vi "Evaluate Method Status.vi"(11 "Results":T2[](array[typedef])) -> (3 "Status":T1)   [LabVIEW 2020, in "Result.lvlib"]
uses:
  Result.lvlib
  Result.ctl
  Status.ctl
  Type.ctl
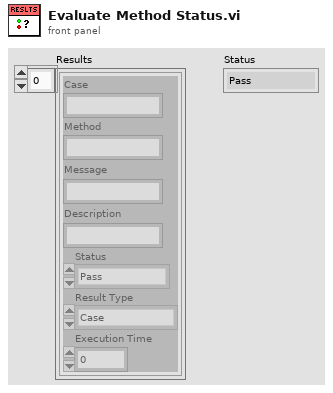
[diagram p1: front panel]
types:
  T1 = typedef "Result.lvlib/Status.ctl" = enum16{"Pass", "Fail", "Error", "Skipped", "Setup Error", "Broken", "Teardown Error"}
  T2 = typedef "Result.lvlib/Result.ctl" = cluster{"Case":string, "Method":string, "Message":string, "Description":string, "Status":T1, "Result Type":T3, "Execution Time":dbl}
  T3 = typedef "Result.lvlib/Type.ctl" = enum16{"Method", "Case", "Suite", "Pass", "Fail", "Skip", "Pass if", "Fail if", "Pass if Error", "Fail if Error", "Pass if Equal", "Fail if Equal"}
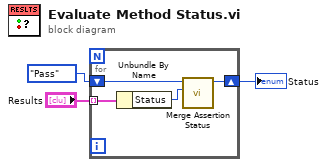
[diagram p0: block diagram]
diagram:
  n1 = for {
    tunnel: "Results" -> [w7] mode=indexing
    shift-right: [w5] -> w1
    shift-left: Status."Pass" ("Current") -> [w6]
    n2 = Unbundle By Name(w7) -> ("Status"=w4:T1)
    n3 = call "Merge Assertion Status.vi"("New"=w4, "Current"=w6) -> ("Merged"=w5:T1)  [unwired: 8 in, 1 out]
  }
  "Status" <- w1
